vi "_PC_Pub_Timestamp_StringTo.vi"(8 "error in":errorcluster, 11 "Timestring":string) -> (0 "error out":errorcluster, 3 "Timestamp":timestamp)   [LabVIEW 2018]
doc: "%I:%M:%S%3u %p%m%d%Y"
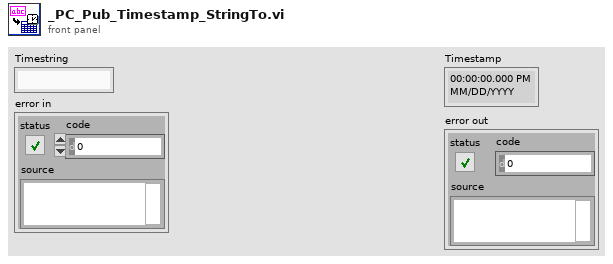
[diagram p1: front panel]
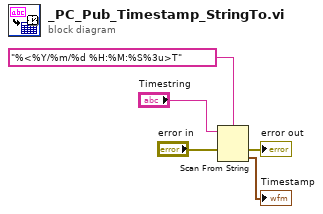
[diagram p0: block diagram]
diagram:
  n1 = Scan From String(format string="%<%Y/%m/%d %H:%M:%S%3u>T", input string="Timestring", error in="error in") -> (error out=→"error out":errorcluster, output 1=→"Timestamp":timestamp)  [unwired: 2 in, 2 out]
